vi "Left Place Beacons (SubVI).vi"(0 "Two Beacons Seen":bool) -> ()   [LabVIEW 2015]
uses:
  Left Variables.vi
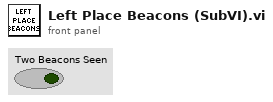
[diagram p1: front panel]
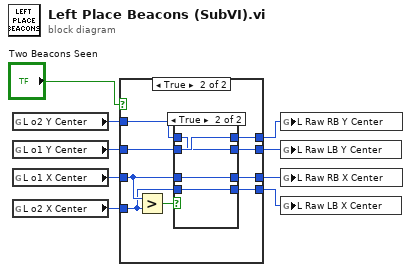
[diagram p0: block diagram]
diagram:
  n1 = global read "Left Variables.vi" "L o2 Y Center"() -> (w1:u16)
  n2 = global read "Left Variables.vi" "L o1 Y Center"() -> (w3:u16)
  n3 = global read "Left Variables.vi" "L o1 X Center"() -> (w4:u16)
  n4 = global read "Left Variables.vi" "L o2 X Center"() -> (w2:u16)
  n5 = case shown="True" "Two Beacons Seen" {
    tunnel: [w10 w20] -> w8
    tunnel: [w10 w19] -> w9
    tunnel: [w11 w18] -> w6
    tunnel: [w11 w17] -> w7
    tunnel: w1 -> [_ w15]
    tunnel: w3 -> [w10 w14]
    tunnel: w4 -> [w11 w13]
    tunnel: w2 -> [_ w12]
    frame False {
    }
    frame True {
      n6 = Greater?(x=w13, y=w12) -> (0:w16:bool)
      n7 = case shown="True" w16 {
        tunnel: w13 -> [w23 w28]
        tunnel: w12 -> [w24 w27]
        tunnel: w14 -> [w21 w26]
        tunnel: w15 -> [w22 w25]
        tunnel: [w24 w28] -> w17
        tunnel: [w23 w27] -> w18
        tunnel: [w22 w26] -> w19
        tunnel: [w21 w25] -> w20
        frame False {
        }
        frame True {
        }
      }
    }
  }
  n8 = global write "Left Variables.vi" "L Raw RB Y Center"(w9) -> ()
  n9 = global write "Left Variables.vi" "L Raw LB Y Center"(w8) -> ()
  n10 = global write "Left Variables.vi" "L Raw RB X Center"(w7) -> ()
  n11 = global write "Left Variables.vi" "L Raw LB X Center"(w6) -> ()
